vi "Publish and Read Back Data.vi"(8 "error in (no error)":errorcluster, 11 "test result id":string) -> (0 "error out":errorcluster, 1 "found hardware items":T4[](array[typedef]), 2 "found software items":T5[](array[typedef]), 3 "queried data":waveform(dbl)(graph), 4 "found operator":T1, 5 "found test station":T3)   [LabVIEW 2024]
uses:
  <vilib>/Plug-In SDKs/Clients/Metadata/Software Item.ctl
  <vilib>/Plug-In SDKs/Clients/Metadata/Extension.ctl
  <vilib>/Plug-In SDKs/Clients/Metadata/Hardware Item.ctl
  <vilib>/Plug-In SDKs/Clients/Metadata/Test Station.ctl
  <vilib>/Plug-In SDKs/Clients/Metadata/Operator.ctl
  <vilib>/Plug-In SDKs/Clients/Metadata/Step.ctl
  <vilib>/Plug-In SDKs/Clients/Data Store V1/Data Store Client.lvlibp/API/Data Store V1/Publish Measurement (DBL Analog Waveform).vi
  <vilib>/Plug-In SDKs/Clients/Data Store V1/Data Store Client.lvlibp/API/Data Store V1/Read Data from Measurement (DBL Analog Waveform).vi
  <vilib>/Plug-In SDKs/Clients/Metadata Store V1/Metadata Store Client.lvlibp/API/Metadata Store V1/Get Test Station.vi
  <vilib>/Plug-In SDKs/Clients/Metadata Store V1/Metadata Store Client.lvlibp/API/Metadata Store V1/Get Hardware Item.vi
  <vilib>/Plug-In SDKs/Clients/Metadata Store V1/Metadata Store Client.lvlibp/API/Metadata Store V1/Get Software Item.vi
  <vilib>/Plug-In SDKs/Clients/Metadata Store V1/Metadata Store Client.lvlibp/API/Metadata Store V1/Get Operator.vi
  <vilib>/Plug-In SDKs/Clients/Data Store V1/Data Store Client.lvlibp
  <vilib>/Plug-In SDKs/Clients/Metadata/NI Metadata Types.lvlib
  <vilib>/measure/NI_MABase.lvlib
  <vilib>/Plug-In SDKs/Clients/Metadata Store V1/Metadata Store Client.lvlibp
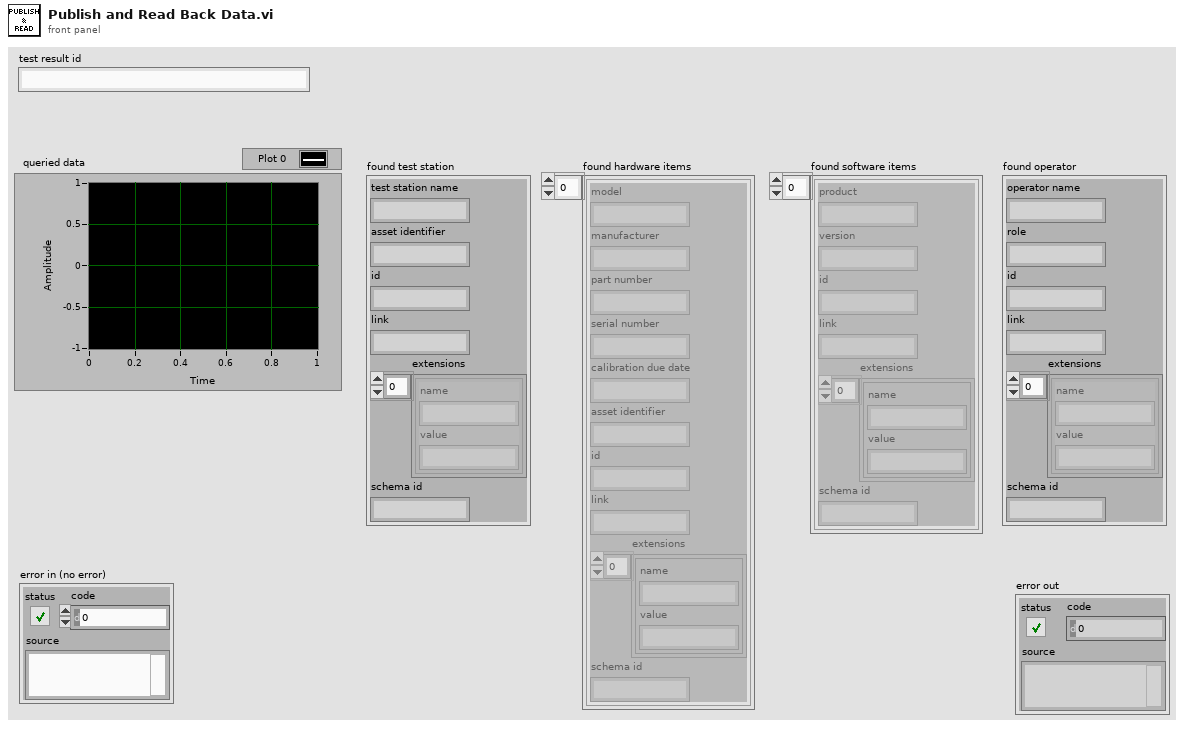
[diagram p1: front panel]
types:
  T1 = typedef "NI Metadata Types.lvlib/Operator.ctl" = cluster{"operator name":string, "role":string, "id":string, "link":string, "extensions":T2[], "schema id":string}
  T2 = typedef "NI Metadata Types.lvlib/Extension.ctl" = cluster{"name":string, "value":string}
  T3 = typedef "NI Metadata Types.lvlib/Test Station.ctl" = cluster{"test station name":string, "asset identifier":string, "id":string, "link":string, "extensions":T2[], "schema id":string}
  T4 = typedef "NI Metadata Types.lvlib/Hardware Item.ctl" = cluster{"model":string, "manufacturer":string, "part number":string, "serial number":string, "calibration due date":string, "asset identifier":string, "id":string, "link":string, "extensions":T2[], "schema id":string}
  T5 = typedef "NI Metadata Types.lvlib/Software Item.ctl" = cluster{"product":string, "version":string, "id":string, "link":string, "extensions":T2[], "schema id":string}
  T6 = typedef "NI Metadata Types.lvlib/Step.ctl" = cluster{"step name":string, "step type":string, "start date time":timestamp, "end date time":timestamp, "notes":string, "step id":string, "parent step id":string, "test result id":string, "test id":string, "link":string, "extensions":T2[], "schema id":string}
  T7 = typedef "Data Store Client.lvlibp/Published Measurement.ctl" = cluster{"data moniker":T8, "published conditions":T9[], "published measurement id":string, "test result id":string, "step id":string, "software item ids":string[], "hardware item ids":string[], "test adapter ids":string[], "measurement name":string, "data type":string, "measurement notes":string, "start date time":timestamp, "end date time":timestamp, "outcome":T10, "parametric index":i32, "error information":T11}
  T8 = typedef "Data Store Client.lvlibp/Data Moniker.ctl" = cluster{"service location":string, "data source":string, "data instance":i64}
  T9 = typedef "Data Store Client.lvlibp/Published Condition.ctl" = cluster{"moniker":T8, "published condition id":string, "condition name":string, "condition type":string, "step id":string, "test result id":string}
  T10 = typedef "NI Metadata Types.lvlib/Outcome.ctl" = enum32{"Unspecified", "Passed", "Failed", "Indeterminate"}
  T11 = typedef "NI Metadata Types.lvlib/Error Information.ctl" = cluster{"error code":i32, "message":string, "source":string}
  T12 = typedef "Data Store Client.lvlibp/Test Result.ctl" = cluster{"test result name":string, "start date time":timestamp, "end date time":timestamp, "outcome":T10, "test result id":string, "uut instance id":string, "operator id":string, "test station id":string, "test description id":string, "software item ids":string[], "hardware item ids":string[], "test adapter ids":string[], "link":string, "extensions":T2[], "schema id":string}
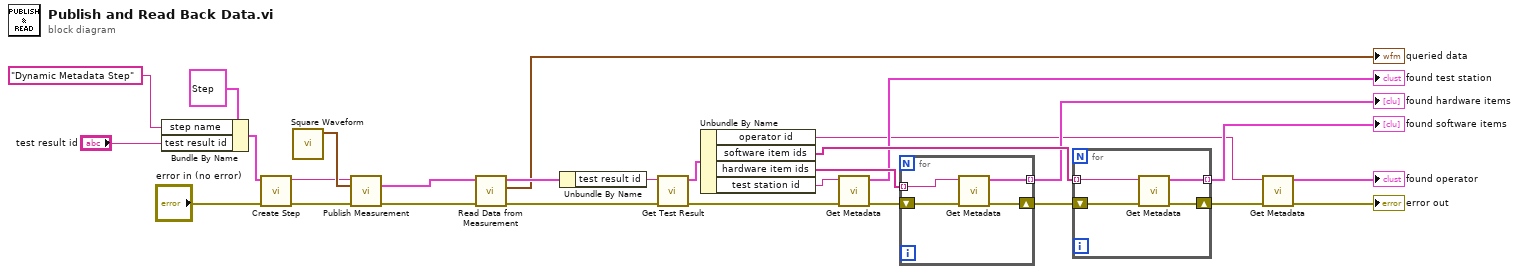
[diagram p0: block diagram]
diagram:
  n1 = Bundle By Name(cluster=T6 {"step name"="", "step type"="", "start date time"=timestamp(0 s since 1904-01-01), "end date time"=timestamp(0 s since 1904-01-01), "notes"="", "step id"="", "parent step id"="", "test result id"="", "test id"="", "link"="", "extensions"=[], "schema id"=""} ("step"), "step name"="Dynamic Metadata Step", "test result id"="test result id") -> (w7:T6)
  n2 = call <vilib>:"Create Step.vi"("error in"="error in (no error)", "step"=w7) -> ("error out"=w10:errorcluster, "step id"=w11:string)  [unwired: 8 in]
  n3 = call <vilib>:"Square Waveform.vi"() -> ("signal out"=w12:waveform(dbl))  [unwired: 10 in, 1 out]
  n4 = call-poly <vilib>:"Publish Measurement.vi"("step id"=w11, "waveform"=w12, "error in"=w10) -> ("published measurement"=w15:T7, "error out"=w13:errorcluster)  [unwired: 10 in, 1 out]
  n5 = call-poly <vilib>:"Read Data from Measurement.vi"("error in"=w13, "published measurement"=w15) -> ("error out"=w17:errorcluster, "waveform data"=→"queried data":waveform(dbl), "published measurement out"=w16:T7)  [unwired: 7 in]
  n6 = Unbundle By Name(w16) -> ("test result id"=w18:string)
  n7 = call <vilib>:"Get Test Result.vi"("error in"=w17, "test result id"=w18) -> ("error out"=w21:errorcluster, "test result"=w19:T12)  [unwired: 8 in]
  n8 = Unbundle By Name(w19) -> ("operator id"=w2:string, "software item ids"=w27:string[], "hardware item ids"=w24:string[], "test station id"=w20:string)
  n9 = call-poly <vilib>:"Get Metadata.vi"("error in"=w21, "test station id"=w20) -> ("error out"=w23:errorcluster, "test station metadata"=→"found test station":T3)  [unwired: 8 in]
  n10 = for {
    shift-right: [w31] -> w26
    shift-left: w23 -> [w32]
    tunnel: w24 -> [w30] mode=indexing
    tunnel: [w29] -> w25 mode=indexing
    n11 = call-poly <vilib>:"Get Metadata.vi"("error in"=w32, "hardware item id"=w30) -> ("error out"=w31:errorcluster, "hardware item"=w29:T4)  [unwired: 8 in]
  }
  "found hardware items" <- w25
  n12 = for {
    shift-right: [w35] -> w4
    shift-left: w26 -> [w36]
    tunnel: w27 -> [w34] mode=indexing
    tunnel: [w33] -> w28 mode=indexing
    n13 = call-poly <vilib>:"Get Metadata.vi"("error in"=w36, "software item id"=w34) -> ("error out"=w35:errorcluster, "software item"=w33:T5)  [unwired: 8 in]
  }
  "found software items" <- w28
  n14 = call-poly <vilib>:"Get Metadata.vi"("error in"=w4, "operator id"=w2) -> ("error out"=→"error out":errorcluster, "operator metadata"=→"found operator":T1)  [unwired: 8 in]
